vi "Global 1.vi"() -> ()   [LabVIEW 2021]
panel:
  out "Blocks Delivered":dbl
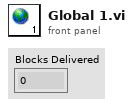
[diagram p1: front panel]
diagram:
